vi "RichToFlatnixnet_grpc_CreateSessionByRefRequest.vi"(5 "OutputClusterType":T1, 11 "InputCluster":T5) -> (3 "OutputCluster":T1)   [LabVIEW 2025, in "grpc-xnet_client.lvlib"]
uses:
  grpc-xnet_client.lvlib
  nixnet_grpc_CreateSessionByRefRequest.ctl
  nixnet_grpc_CreateSessionByRefRequest_mode_enum/nixnet_grpc_CreateSessionByRefRequest_mode_enum.lvclass
  nidevice_grpc_Session.ctl
  nidevice_grpc_SessionInitializationBehavior.ctl
  nixnet_grpc_CreateSessionByRefRequest_Flat.ctl
  nidevice_grpc_Session_Flat.ctl
  nixnet_grpc_CreateSessionMode.ctl
  nixnet_grpc_CreateSessionByRefRequest_mode_enum/nixnet_grpc_CreateSessionByRefRequest_mode_enum.lvclass/nixnet_grpc_CreateSessionByRefRequest_mode_enum.ctl
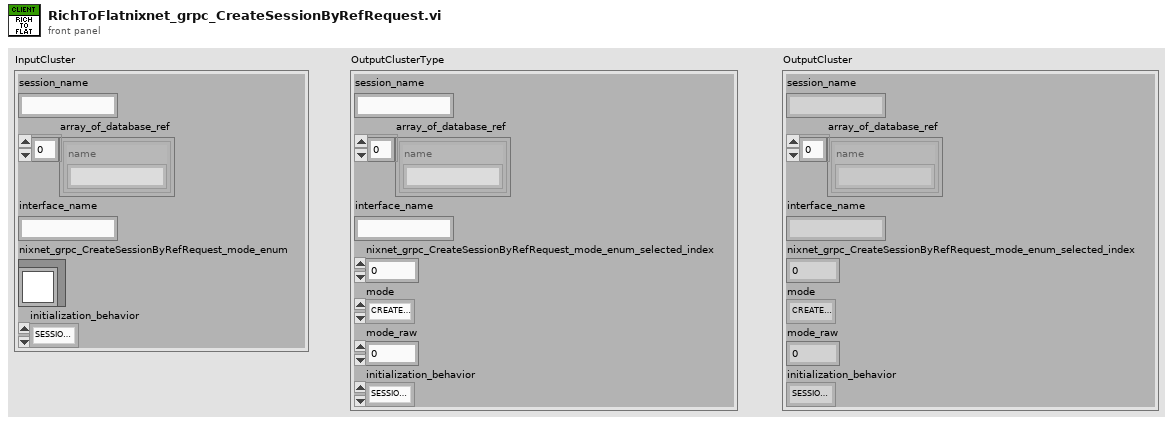
[diagram p1: front panel]
types:
  T1 = typedef "grpc-xnet_client.lvlib/nixnet_grpc_CreateSessionByRefRequest_Flat.ctl" = cluster{"session_name":string, "array_of_database_ref":T2[], "interface_name":string, "nixnet_grpc_CreateSessionByRefRequest_mode_enum_selected_index":i32, "mode":T3, "mode_raw":u32, "initialization_behavior":T4}
  T2 = typedef "grpc-xnet_client.lvlib/nidevice_grpc_Session_Flat.ctl" = cluster{"name":string}
  T3 = typedef "grpc-xnet_client.lvlib/nixnet_grpc_CreateSessionMode.ctl" = enum32{"CREATE_SESSION_MODE_SIGNAL_IN_SINGLE_POINT", "CREATE_SESSION_MODE_SIGNAL_IN_WAVEFORM", "CREATE_SESSION_MODE_SIGNAL_IN_XY", "CREATE_SESSION_MODE_SIGNAL_OUT_SINGLE_POINT", "CREATE_SESSION_MODE_SIGNAL_OUT_WAVEFORM", "CREATE_SESSION_MODE_SIGNAL_OUT_XY", "CREATE_SESSION_MODE_FRAME_IN_STREAM", "CREATE_SESSION_MODE_FRAME_IN_QUEUED", "CREATE_SESSION_MODE_FRAME_IN_SINGLE_POINT", "CREATE_SESSION_MODE_FRAME_OUT_STREAM", "CREATE_SESSION_MODE_FRAME_OUT_QUEUED", "CREATE_SESSION_MODE_FRAME_OUT_SINGLE_POINT", "CREATE_SESSION_MODE_SIGNAL_CONVERSION_SINGLE_POINT"}
  T4 = typedef "grpc-xnet_client.lvlib/nidevice_grpc_SessionInitializationBehavior.ctl" = enum32{"SESSION_INITIALIZATION_BEHAVIOR_UNSPECIFIED", "SESSION_INITIALIZATION_BEHAVIOR_INITIALIZE_NEW", "SESSION_INITIALIZATION_BEHAVIOR_ATTACH_TO_EXISTING"}
  T5 = typedef "grpc-xnet_client.lvlib/nixnet_grpc_CreateSessionByRefRequest.ctl" = cluster{"session_name":string, "array_of_database_ref":T6[], "interface_name":string, "nixnet_grpc_CreateSessionByRefRequest_mode_enum":refnum<class "nixnet_grpc_CreateSessionByRefRequest_mode_enum.lvclass">, "initialization_behavior":T4}
  T6 = typedef "grpc-xnet_client.lvlib/nidevice_grpc_Session.ctl" = cluster{"name":string}
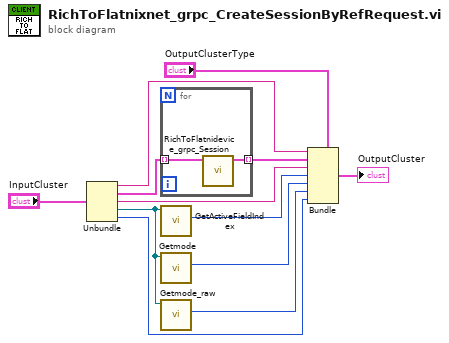
[diagram p0: block diagram]
diagram:
  n1 = Unbundle "Unbundle"("InputCluster") -> ("session_name"=w9:string, "array_of_database_ref"=w8:T6[], "interface_name"=w6:string, "nixnet_grpc_CreateSessionByRefRequest_mode_enum"=w5:refnum<class "nixnet_grpc_CreateSessionByRefRequest_mode_enum.lvclass">, "initialization_behavior"=w1:T4)
  n2 = for {
    tunnel: w8 -> [w14] mode=indexing
    tunnel: [w13] -> w7 mode=indexing
    n3 = call "RichToFlatnidevice_grpc_Session.vi"("InputCluster"=w14) -> ("OutputCluster"=w13:T2)  [unwired: 10 in]
  }
  n4 = call "GetActiveFieldIndex.vi"("OneOfTemplate in"=w5) -> ("Active Field Index"=w4:i32)  [unwired: 8 in, 2 out]
  n5 = call "Getmode.vi"("OneOfTemplate in"=w5) -> ("Get_Val"=w3:T3)  [unwired: 8 in, 2 out]
  n6 = call "Getmode_raw.vi"("OneOfTemplate in"=w5) -> ("Get_Val"=w2:u32)  [unwired: 8 in, 2 out]
  n7 = Bundle "Bundle"(cluster="OutputClusterType", "session_name"=w9, "array_of_database_ref"=w7, "interface_name"=w6, "nixnet_grpc_CreateSessionByRefRequest_mode_enum_selected_index"=w4, "mode"=w3, "mode_raw"=w2, "initialization_behavior"=w1) -> (→"OutputCluster":T1)
